vi "NotifyWithoutDataOverride.vi"(8 "error in (no error)":errorcluster, 11 "Normal Com in":refnum<class "Normal Com.lvclass">) -> (0 "error out":errorcluster, 2 "Data out":refnum<class "Data.lvclass">, 3 "Normal Com out":refnum<class "Normal Com.lvclass">)   [LabVIEW 2023, in "Normal Com.lvclass"]
uses:
  Normal Com.lvclass
  C:/Users/santharu.subramanian/Desktop/LOA New/Documents/LV New Assignments/Sender-Receiver/Classes/Communication/Communication.lvclass
  Data/Data.lvclass
  Normal Com.lvclass/Normal Com.ctl
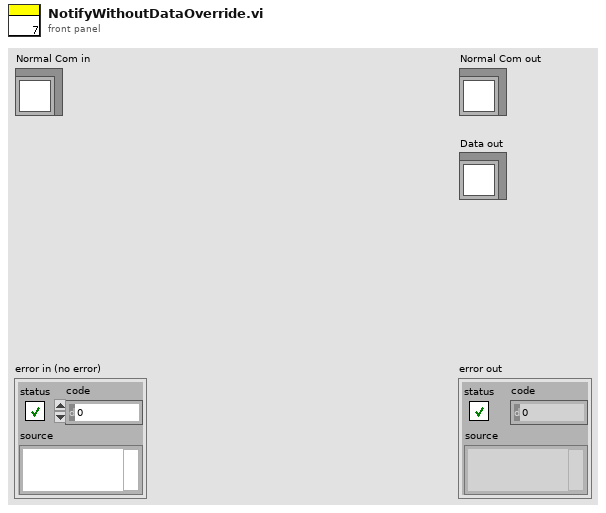
[diagram p1: front panel]
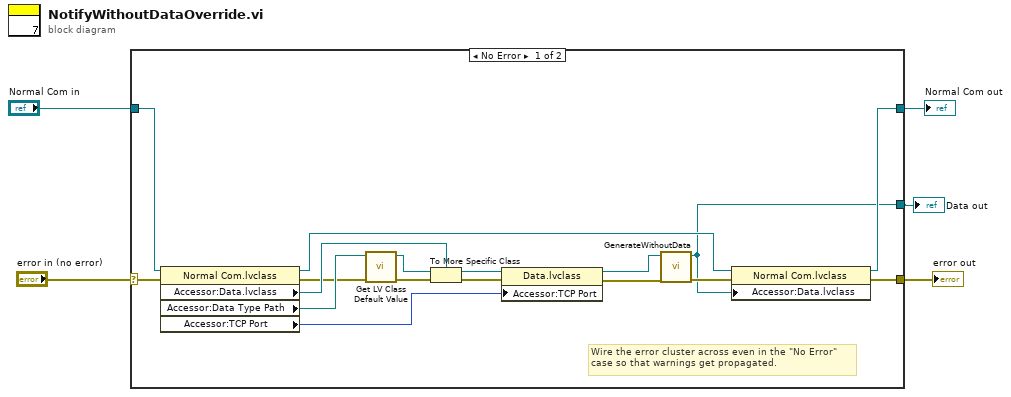
[diagram p0: block diagram]
diagram:
  n1 = case shown="No Error" "error in (no error)" {
    selector: "error in (no error)" -> [w22 w24]
    tunnel: [w13 w24] -> w4
    tunnel: [w11 w23] -> w2
    tunnel: "Normal Com in" -> [w21 w23]
    tunnel: [w10 _] -> w1
    frame No Error {
      # "Wire the error cluster across even in the \"No Error\"\ncase so that warnings get propagated."
      n2 = property class="Normal Com.lvclass"(reference=w21, error in=w22) -> (reference out=w12:refnum<class "Normal Com.lvclass">, error out=w15:errorcluster, "Accessor:Data.lvclass"=w17:refnum<class "Data.lvclass">, "Accessor:Data Type Path"=w16:path, "Accessor:TCP Port"=w6:u16)
      n3 = call <vilib>:"Get LV Class Default Value.vi"("error in (no error)"=w15, "class path"=w16) -> ("error out"=w20:errorcluster, "object"=w19:refnum<class>)  [unwired: 8 in]
      n4 = To More Specific Class(target class=w17, reference=w19, error in=w20) -> (specific class reference=w18:refnum<class "Data.lvclass">, error out=w8:errorcluster)
      n5 = property class="Data.lvclass"(reference=w18, error in=w8, "Accessor:TCP Port"=w6) -> (reference out=w9:refnum<class "Data.lvclass">, error out=w7:errorcluster)
      n6 = call-dynamic "GenerateWithoutData.vi"("error in (no error)"=w7, "Data in"=w9) -> ("error out"=w14:errorcluster, "Data out"=w10:refnum<class "Data.lvclass">)  [unwired: 8 in]
      n7 = property class="Normal Com.lvclass"(reference=w12, error in=w14, "Accessor:Data.lvclass"=w10) -> (reference out=w11:refnum<class "Normal Com.lvclass">, error out=w13:errorcluster)
    }
    frame Error {
    }
  }
  "error out" <- w4
  "Normal Com out" <- w2
  "Data out" <- w1
